vi "Logging Message Loop.vi"(8 "error in (no error)":errorcluster, 10 "Data Queue":refnum<queue>, 11 "Message Queues":T1) -> (0 "error out":errorcluster)   [LabVIEW 2018, in "Logging.lvlib"]
doc: "The message loop subVI to handle messages pertaining to logging data."
uses:
  Logging.lvlib
  support/Message Queue/All Message Queues.ctl
  support/Message Queue/Message Cluster.ctl
  Logging Configuration.ctl
  Logging State.ctl
  support/Message Queue/Enqueue Message (Single).vi
  <vilib>/Utility/error.llb/Error Cluster From Error Code.vi
  <vilib>/ErrorRing/Error Ring.xnode
  support/Message Queue/Message Queue.lvlib
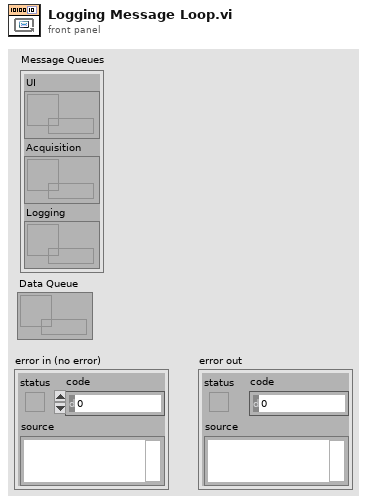
[diagram p1: front panel]
types:
  T1 = typedef "Message Queue.lvlib/All Message Queues.ctl" = cluster{"UI":refnum<queue>, "Acquisition":refnum<queue>, "Logging":refnum<queue>}
  T2 = typedef "Logging.lvlib/Logging Configuration.ctl" = cluster{"Log File Base Path":path, "TDMS File Reference":refnum<k34>}
  T3 = typedef "Logging.lvlib/Logging State.ctl" = enum16{"Idle", "Logging"}
  T4 = enum16{"open", "open or create", "create or replace", "create", "open (read-only)"}
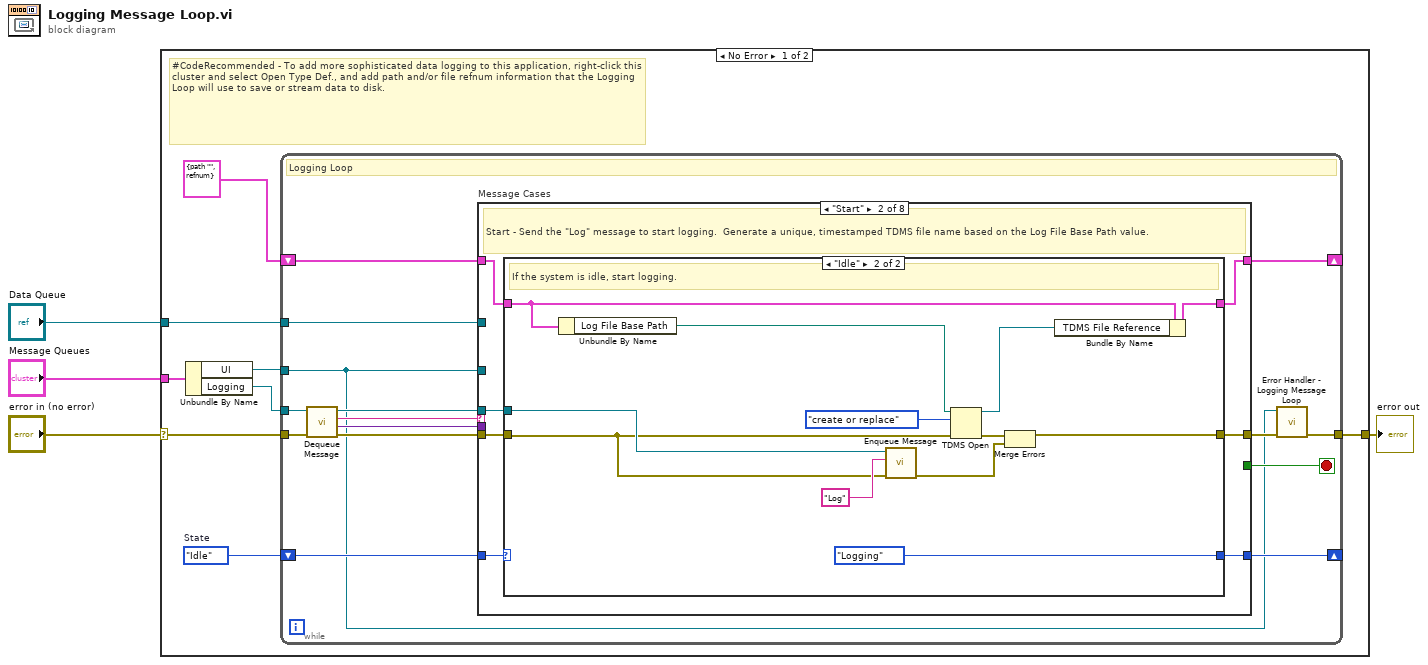
[diagram p0: block diagram]
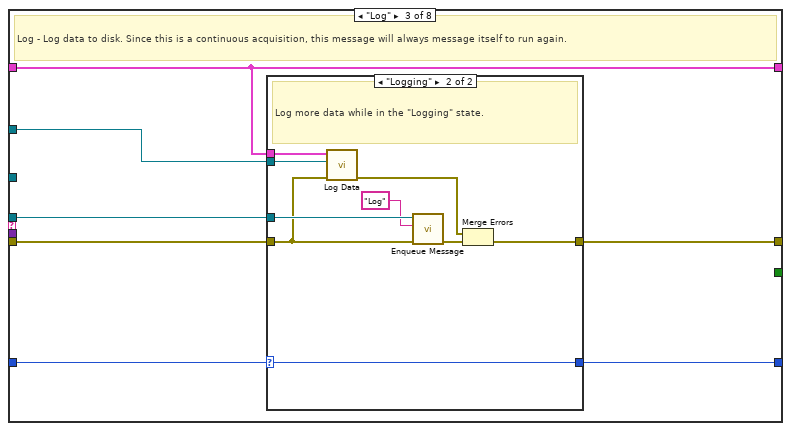
[diagram p4: hidden frame]
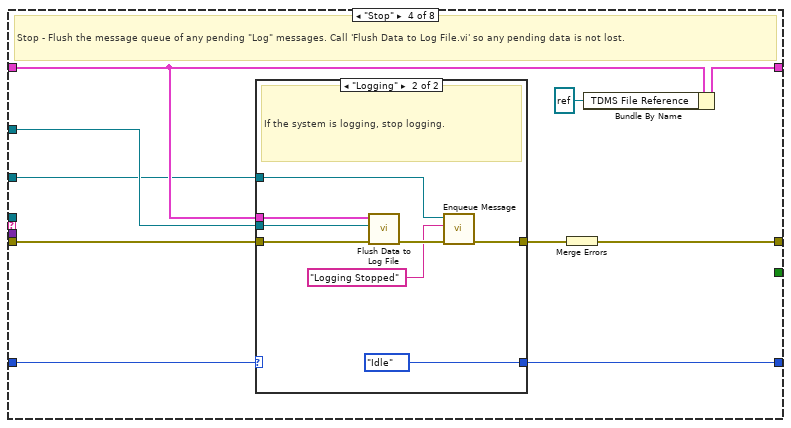
[diagram p6: hidden frame]
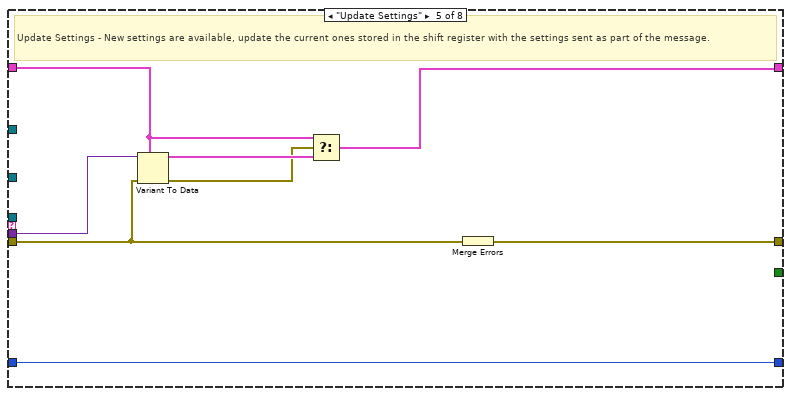
[diagram p8: hidden frame]
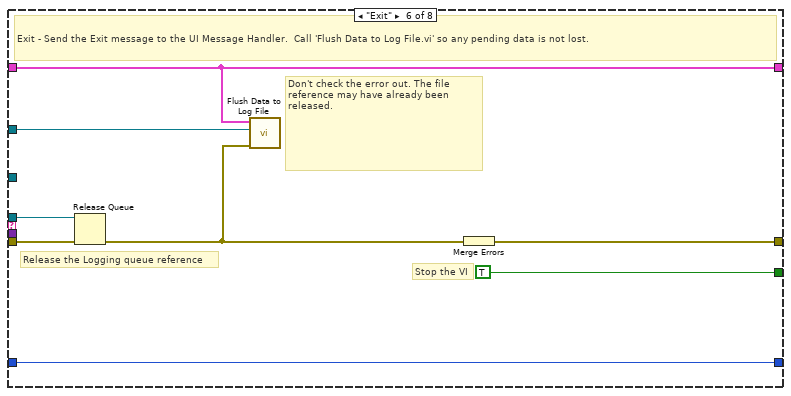
[diagram p9: hidden frame]
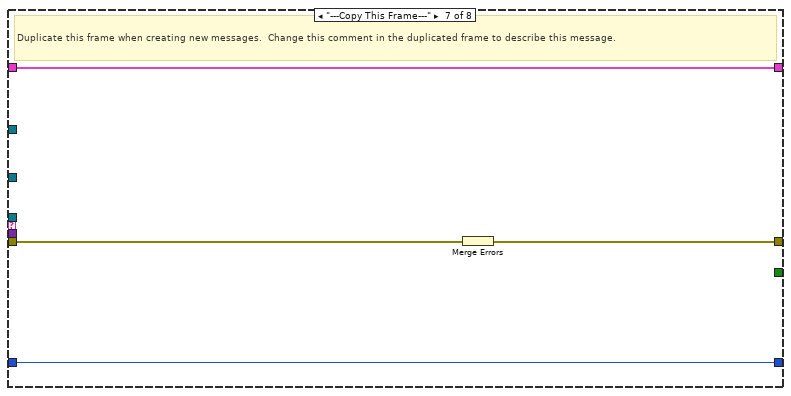
[diagram p10: hidden frame]
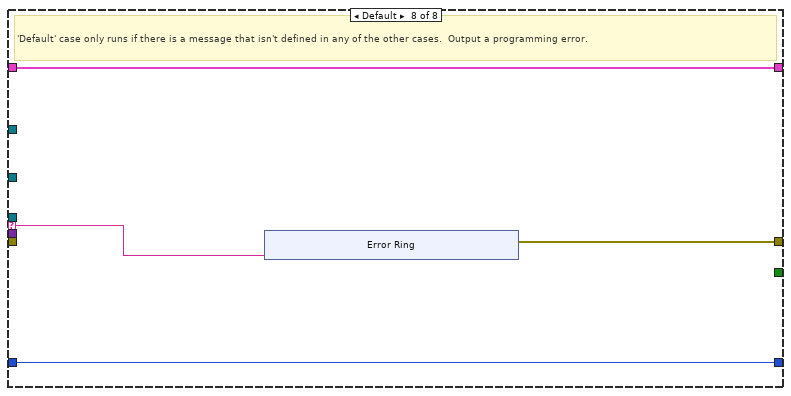
[diagram p11: hidden frame]
diagram:
  n1 = case shown="No Error" "error in (no error)" {
    selector: "error in (no error)" -> [w8 w122]
    tunnel: "Message Queues" -> [w12 _]
    tunnel: [w10 w122] -> w3
    tunnel: "Data Queue" -> [w7 _]
    frame No Error {
      w5 = Logging_State."Idle"  # State
      # "#CodeRecommended - To add more sophisticated data logging to this application, right-click this cluster and select Open Type Def., and add path and/or file refnum information that the Logging Loop will use to save or stream data to disk."
      n2 = Unbundle By Name(w12) -> ("UI"=w6:refnum<queue>, "Logging"=w11:refnum<queue>)
      n3 = while {
        tunnel: w11 -> [w19]
        shift-right: [w26] -> _
        shift-left: T2 {"Log File Base Path"=path "", "TDMS File Reference"=refnum} ("Logging Configuration") -> [w27]
        tunnel: w6 -> [w13]
        tunnel: w7 -> [w18]
        shift-right: [w16] -> _
        shift-left: w5 -> [w17]
        tunnel: w8 -> [w24]
        tunnel: [w15] -> w10
        stop <- w25 stop-if-true
        # "Logging Loop"
        n4 = call "Dequeue Message.vi"("error in (no error)"=w24, "Message Queue"=w19) -> ("error out"=w23:errorcluster, "Message Data"=w21:variant, "Message"=w22:string, "dup Message Queue"=w20:refnum<queue>)  [unwired: 6 in]
        n5 = case "Message Cases" shown="\"Start\"" w22 {
          selector: w22 -> [_ _ _ _ _ _ _ w111]
          tunnel: w20 -> [_ w36 w58 _ _ w103 _ _]
          tunnel: w23 -> [w29 w35 w56 w74 w92 w104 w110 _]
          tunnel: [w29 w37 w59 w80 w98 w105 w108 w112] -> w14
          tunnel: w27 -> [w30 w34 w55 w75 w96 w101 w109 w114]
          tunnel: [w30 w33 w55 w78 w93 w101 w109 w114] -> w26
          tunnel: [_ _ _ _ _ TRUE _ _] -> w25
          tunnel: w21 -> [_ _ _ _ w97 _ _ _]
          tunnel: w13 -> [_ _ _ w71 _ _ _ _]
          tunnel: w18 -> [_ _ w57 w76 _ w100 _ _]
          tunnel: w17 -> [w28 w32 w54 w73 w91 w99 w107 w113]
          tunnel: [w28 w31 w53 w72 w91 w99 w107 w113] -> w16
          frame "Initialize" {
            # "Initialize - gets called when first launched. Currently a no-op."
          }
          frame "Start" {
            # "Start - Send the \"Log\" message to start logging.  Generate a unique, timestamped TDMS file name based on the Log File Base Path value."
            n6 = case shown="\"Idle\"" w32 {
              selector: w32 -> [w39 _]
              tunnel: [w38 w43] -> w37
              tunnel: w36 -> [_ w44]
              tunnel: w35 -> [w38 w42]
              tunnel: w34 -> [w40 w45]
              tunnel: [w40 w47] -> w33
              tunnel: [w39 Logging_State."Logging" ("State")] -> w31
              frame "Logging" {
                # "The system is already logging. Ignore the \"Start\" message."
              }
              frame "Idle" {
                # "If the system is idle, start logging."
                n7 = Unbundle By Name(w45) -> ("Log File Base Path"=w41:path)
                n8 = call-poly "Enqueue Message.vi"("error in (no error)"=w42, "Message"="Log", "Message Queue"=w44) -> ("error out"=w50:errorcluster)  [unwired: 7 in, 1 out]
                n9 = TDMS Open(8:w42, 10:T4."create or replace" ("operation (0:open)"), 11:w41) -> (0:w51:errorcluster, 3:w48:refnum<k34>)  [unwired: 4 in]
                n10 = Merge Errors(w51, w50) -> (w43:errorcluster)
                n11 = Bundle By Name(cluster=w45, "TDMS File Reference"=w48) -> (w47:T2)
              }
            }
          }
          frame "Log" {
            # "Log - Log data to disk. Since this is a continuous acquisition, this message will always message itself to run again."
            n12 = case shown="\"Logging\"" w54 {
              selector: w54 -> [w61 w63]
              tunnel: [w60 w70] -> w59
              tunnel: w58 -> [_ w68]
              tunnel: w57 -> [_ w67]
              tunnel: w56 -> [w60 w62]
              tunnel: w55 -> [_ w64]
              tunnel: [w61 w63] -> w53
              frame "Idle" {
                # "Ignore \"Log\" messages when the logging is idle."
              }
              frame "Logging" {
                # "Log more data while in the \"Logging\" state."
                n13 = call "Log Data.vi"("error in (no error)"=w62, "Data Queue"=w67, "Logging Configuration"=w64) -> ("error out"=w66:errorcluster)  [unwired: 8 in]
                n14 = call-poly "Enqueue Message.vi"("error in (no error)"=w62, "Message"="Log", "Message Queue"=w68) -> ("error out"=w69:errorcluster)  [unwired: 7 in, 1 out]
                n15 = Merge Errors(w66, w69) -> (w70:errorcluster)
              }
            }
          }
          frame "Stop" {
            # "Stop - Flush the message queue of any pending \"Log\" messages. Call 'Flush Data to Log File.vi' so any pending data is not lost."
            n16 = case shown="\"Logging\"" w73 {
              selector: w73 -> [w81 _]
              tunnel: [w82 w85] -> w79
              tunnel: w76 -> [_ w89]
              tunnel: w75 -> [_ w88]
              tunnel: w74 -> [w82 w87]
              tunnel: [w81 Logging_State."Idle" ("State")] -> w72
              tunnel: w71 -> [_ w84]
              frame "Idle" {
                # "The system is already idle. Ignore the \"Stop\" message."
              }
              frame "Logging" {
                # "If the system is logging, stop logging."
                n17 = call "Flush Data to Log File.vi"("error in (no error)"=w87, "Data Queue"=w89, "Logging Configuration"=w88) -> ("error out"=w90:errorcluster)  [unwired: 8 in]
                n18 = call-poly "Enqueue Message.vi"("error in (no error)"=w90, "Message"="Logging Stopped", "Message Queue"=w84) -> ("error out"=w85:errorcluster)  [unwired: 7 in, 1 out]
              }
            }
            n19 = Merge Errors(w79) -> (w80:errorcluster)
            n20 = Bundle By Name(cluster=w75, "TDMS File Reference"=refnum<k34> refnum) -> (w78:T2)
          }
          frame "Update Settings" {
            # "Update Settings - New settings are available, update the current ones stored in the shift register with the settings sent as part of the message."
            n21 = Variant To Data(error in=w92, type=w96, Variant=w97) -> (data=w95:T2, error out=w94:errorcluster)
            n22 = Select(t=w96, s=w94, f=w95) -> (s? t:f=w93:T2)
            n23 = Merge Errors(w92) -> (w98:errorcluster)
          }
          frame "Exit" {
            # "Don't check the error out. The file reference may have already been released."
            # "Release the Logging queue reference"
            # "Stop the VI"
            # "Exit - Send the Exit message to the UI Message Handler.  Call 'Flush Data to Log File.vi' so any pending data is not lost."
            n24 = Release Queue(queue=w103, error in (no error)=w104) -> (error out=w102:errorcluster)  [unwired: 1 in, 2 out]
            n25 = call "Flush Data to Log File.vi"("error in (no error)"=w102, "Data Queue"=w100, "Logging Configuration"=w101) -> ()  [unwired: 8 in, 1 out]
            n26 = Merge Errors(w102) -> (w105:errorcluster)
          }
          frame "---Copy This Frame---" {
            # "Duplicate this frame when creating new messages.  Change this comment in the duplicated frame to describe this message."
            n27 = Merge Errors(w110) -> (w108:errorcluster)
          }
          frame Default {
            # "'Default' case only runs if there is a message that isn't defined in any of the other cases.  Output a programming error."
            n28 = xnode "Error Ring"("parameter 0"=w111) -> ("error out"=w112:errorcluster)
          }
        }
        n29 = call "Error Handler - Logging Message Loop.vi"("error in (no error)"=w14, "Message Queue"=w13) -> ("dup error in"=w15:errorcluster)  [unwired: 8 in, 1 out]
      }
    }
    frame Error {
    }
  }
  "error out" <- w3
